vi "main.vi"() -> ()   [LabVIEW 2013]
uses:
  <vilib>/Utility/error.llb/DialogType.ctl
panel:
  out "con status":bool
  in  "Autoscale":bool=TRUE
  in  "P max":dbl=300.0 min=2.0 max=500.0 step=0.1
  in  "P min":dbl=4.0 min=-10.0 max=350.0 step=0.1
  in  "ВКЛ/ВЫКЛ 4":bool=TRUE
  in  "ВКЛ/ВЫКЛ 3":bool=TRUE
  in  "ВКЛ/ВЫКЛ 2":bool
  in  "ВКЛ/ВЫКЛ 1":bool=TRUE
  out "B2":string
  out "B1":string
  out "A2":string
  out "A1":string
  in  "remote port":u16=4001
  in  "address":string="192.168.127.253"
  in  "xScale +":bool
  in  "xScale -":bool
  in  "Добавить время":dbl(ring)=300.0 items=["1 мин."=60.0, "5 мин."=300.0, "20 мин."=1200.0]
  out "мин.":string="1"
  out "часы":string="0"
  out "Graphs hP":dynamicdata(graph) caption="Высокий вакуум, мБар"
  out "сек.":string="0"
  out "Сутки":string
  out "Graphs lP":dynamicdata(graph) caption="Низкий вакуум, мБар"
  in  "stop":bool
  # "Интервал просмотра"
  # ":"
types:
  T1 = typedef "DialogType.ctl" = u16
  T2 = typedef "LVDateTimeRec.ctl" = cluster{"fractional second":dbl, "second":i32, "minute":i32, "hour":i32, "day of month":i32, "month":i32, "year":i32, "day of week":i32, "day of year":i32, "DST":i32}
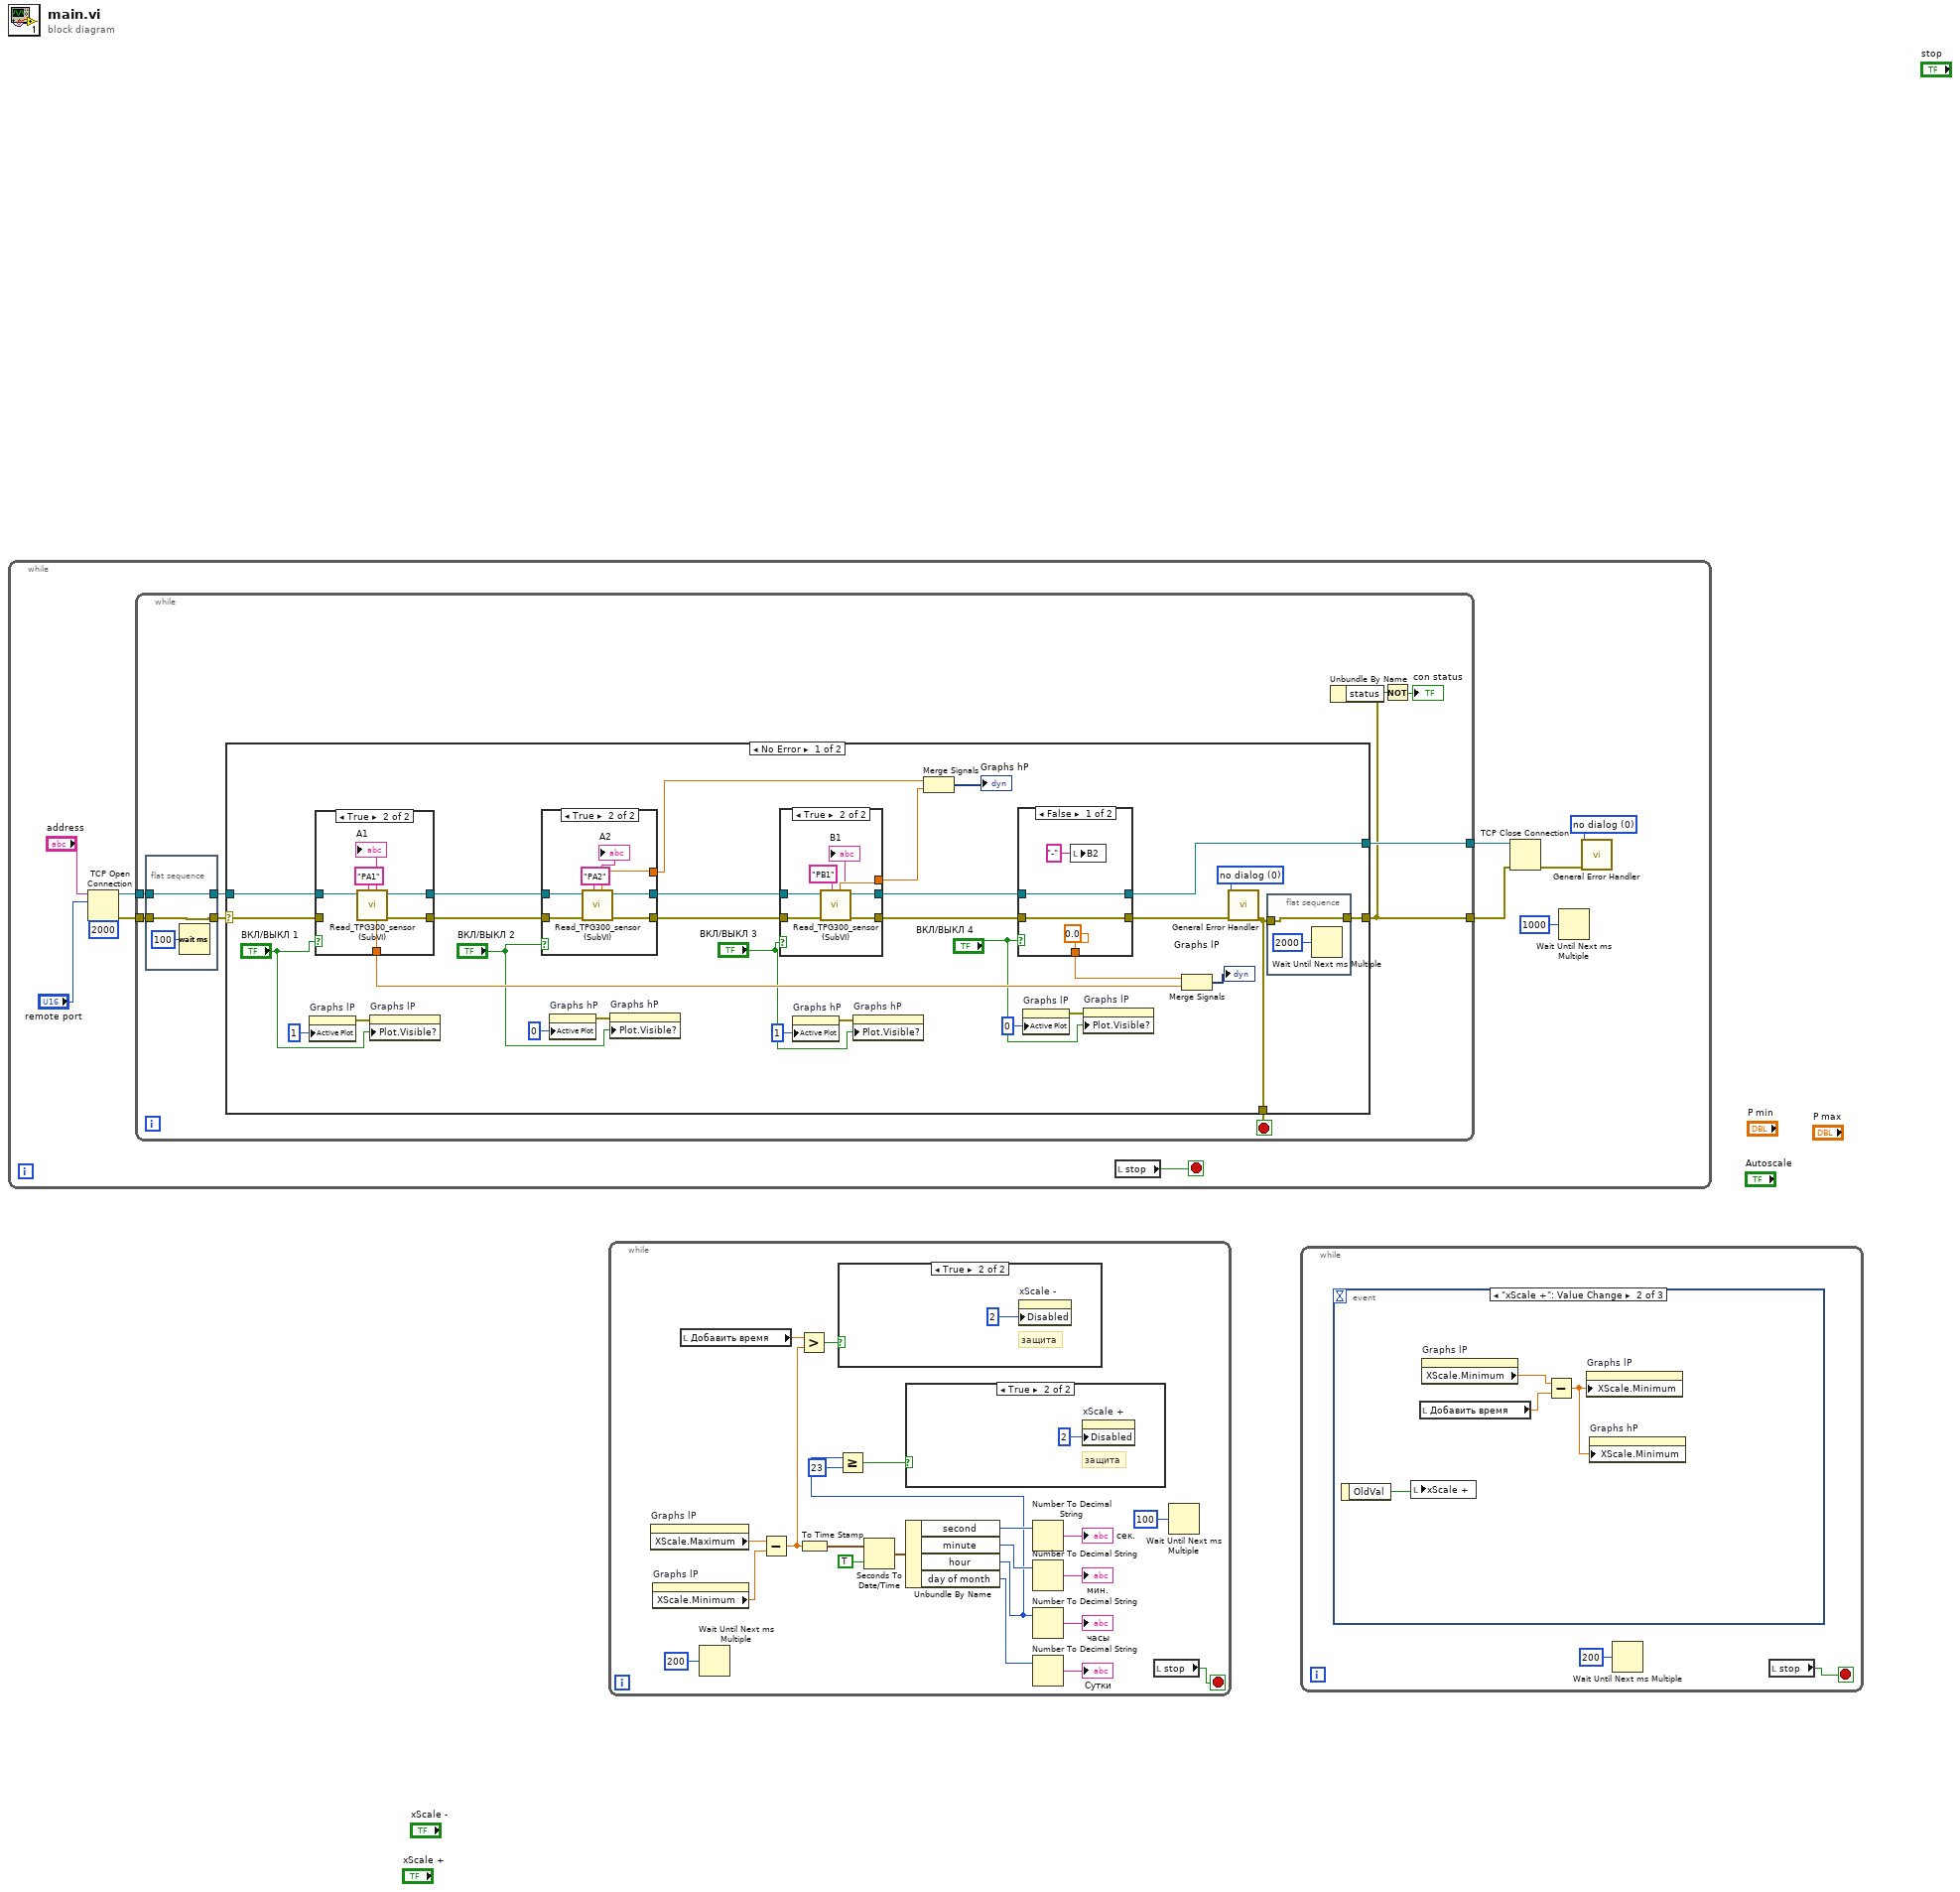
[diagram p0: block diagram]
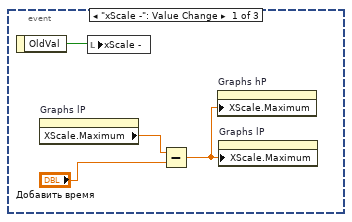
[diagram p2: hidden frame]
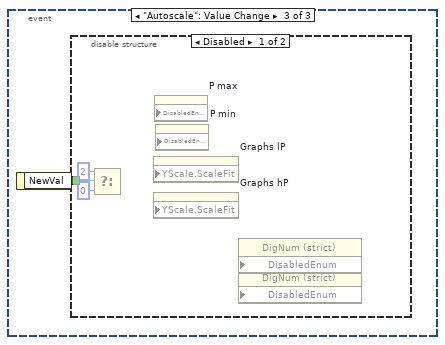
[diagram p3: hidden frame]
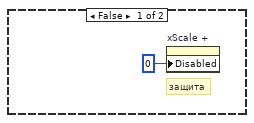
[diagram p5: hidden frame]
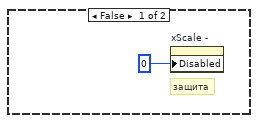
[diagram p6: hidden frame]
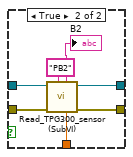
[diagram p7: hidden frame]
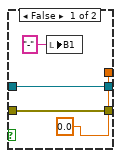
[diagram p8: hidden frame]
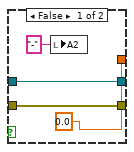
[diagram p9: hidden frame]
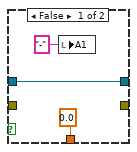
[diagram p10: hidden frame]
diagram:
  n1 = while {
    stop <- w11 stop-if-true
    w5 = T1 0 items=["no dialog", "OK message", "continue or stop message", "OK message + warnings", "continue/stop + warnings"] ("type of dialog (OK msg:1)")
    n2 = TCP Open Connection(address="address", remote port or service name="remote port", timeout ms (60000)=2000) -> (connection ID=w9:refnum<k5>, error out=w8:errorcluster)  [unwired: 1 in, 1 out]
    n3 = while {
      tunnel: w9 -> [w18]
      tunnel: w8 -> [w15]
      tunnel: [w19] -> w6
      tunnel: [w14] -> w3
      stop <- w20 stop-if-true
      n4 = flat-sequence {
        tunnel: w18 -> [w23]
        tunnel: [w23] -> w17
        tunnel: [w22] -> w16
        tunnel: w15 -> [w22]
        frame #0 {
          n5 = Wait (ms)(milliseconds to wait=u32 100) -> ()  [unwired: 1 out]
        }
      }
      n6 = case shown="No Error" w16 {
        selector: w16 -> [w54 w99]
        tunnel: w17 -> [w53 w100]
        tunnel: [w29 w99] -> w20
        tunnel: [w43 w100] -> w19
        tunnel: [w28 w99] -> w14
        frame No Error {
          w44 = T1 0 items=["no dialog", "OK message", "continue or stop message", "OK message + warnings", "continue/stop + warnings"] ("type of dialog (OK msg:1)")
          n7 = property on="Graphs lP" class="WFChart (strict)"("Active Plot"=u32 1) -> (error out=w40:errorcluster)  [unwired: 2 in, 1 out]
          n8 = case shown="True" "ВКЛ/ВЫКЛ 1" {
            tunnel: w54 -> [_ _]
            tunnel: w53 -> [w92 w98]
            tunnel: [_ w96] -> w52
            tunnel: [w92 w95] -> w51
            tunnel: [0.0 ("out number") w94] -> w50
            frame False {
              n9 = local write "A1"("-" ("A1")) -> ()
            }
            frame True {
              n10 = call "Read_TPG300_sensor (SubVI).vi"("Sensor CMD"="PA1" ("data in"), "TCP Network Connection in"=w98) -> ("error out"=w96:errorcluster, "connection ID out"=w95:refnum<k5>, "out number"=w94:dbl, "data out"=→"A1":string)  [unwired: 6 in]
            }
          }
          n11 = property on="Graphs lP" class="WFChart (strict)"(error in=w40, "Plot.Visible?"="ВКЛ/ВЫКЛ 1") -> ()  [unwired: 1 in, 2 out]
          n12 = case shown="True" "ВКЛ/ВЫКЛ 2" {
            tunnel: w52 -> [w81 w89]
            tunnel: w51 -> [w82 w88]
            tunnel: [w82 w87] -> w48
            tunnel: [w81 w86] -> w49
            tunnel: [0.0 ("out number") w84] -> w26
            frame False {
              n13 = local write "A2"("-" ("A2")) -> ()
            }
            frame True {
              n14 = call "Read_TPG300_sensor (SubVI).vi"("Sensor CMD"="PA2" ("data in"), "error in (no error)"=w89, "TCP Network Connection in"=w88) -> ("error out"=w86:errorcluster, "connection ID out"=w87:refnum<k5>, "out number"=w84:dbl, "data out"=→"A2":string)  [unwired: 5 in]
            }
          }
          n15 = property on="Graphs hP" class="WFChart (strict)"("Active Plot"=u32 0) -> (error out=w38:errorcluster)  [unwired: 2 in, 1 out]
          n16 = property on="Graphs hP" class="WFChart (strict)"(error in=w38, "Plot.Visible?"="ВКЛ/ВЫКЛ 2") -> ()  [unwired: 1 in, 2 out]
          n17 = case shown="True" "ВКЛ/ВЫКЛ 3" {
            tunnel: w49 -> [w70 w77]
            tunnel: w48 -> [w71 w76]
            tunnel: [w70 w75] -> w47
            tunnel: [w71 w74] -> w46
            tunnel: [0.0 ("out number") w73] -> w25
            frame False {
              n18 = local write "B1"("-" ("B1")) -> ()
            }
            frame True {
              n19 = call "Read_TPG300_sensor (SubVI).vi"("Sensor CMD"="PB1" ("data in"), "error in (no error)"=w77, "TCP Network Connection in"=w76) -> ("error out"=w75:errorcluster, "connection ID out"=w74:refnum<k5>, "out number"=w73:dbl, "data out"=→"B1":string)  [unwired: 5 in]
            }
          }
          n20 = property on="Graphs hP" class="WFChart (strict)"("Active Plot"=u32 1) -> (error out=w34:errorcluster)  [unwired: 2 in, 1 out]
          n21 = property on="Graphs hP" class="WFChart (strict)"(error in=w34, "Plot.Visible?"="ВКЛ/ВЫКЛ 3") -> ()  [unwired: 1 in, 2 out]
          n22 = Merge Signals(w26, w25) -> (→"Graphs hP":dynamicdata)
          n23 = case shown="False" "ВКЛ/ВЫКЛ 4" {
            tunnel: w47 -> [w60 w66]
            tunnel: w46 -> [w59 w65]
            tunnel: [0.0 ("out number") w64] -> w27
            tunnel: [w60 w63] -> w45
            tunnel: [w59 w62] -> w43
            frame False {
              n24 = local write "B2"("-" ("B2")) -> ()
            }
            frame True {
              n25 = call "Read_TPG300_sensor (SubVI).vi"("Sensor CMD"="PB2" ("data in"), "error in (no error)"=w66, "TCP Network Connection in"=w65) -> ("error out"=w63:errorcluster, "connection ID out"=w62:refnum<k5>, "out number"=w64:dbl, "data out"=→"B2":string)  [unwired: 5 in]
            }
          }
          n26 = property on="Graphs lP" class="WFChart (strict)"("Active Plot"=u32 0) -> (error out=w32:errorcluster)  [unwired: 2 in, 1 out]
          n27 = property on="Graphs lP" class="WFChart (strict)"(error in=w32, "Plot.Visible?"="ВКЛ/ВЫКЛ 4") -> ()  [unwired: 1 in, 2 out]
          n28 = Merge Signals(w27, w50) -> (→"Graphs lP":dynamicdata)
          n29 = call <vilib>:"General Error Handler.vi"("type of dialog (OK msg:1)"=w44, "error in (no error)"=w45) -> ("error out"=w29:errorcluster)  [unwired: 9 in, 4 out]
          n30 = flat-sequence {
            tunnel: w29 -> [w55]
            tunnel: [w55] -> w28
            frame #0 {
              n31 = Wait Until Next ms Multiple(millisecond multiple=u32 2000) -> ()  [unwired: 1 out]
            }
          }
        }
        frame Error {
        }
      }
      n32 = Unbundle By Name(w14) -> ("status"=w13:bool)
      n33 = Not(x=w13) -> (.not. x?=→"con status":bool)
    }
    n34 = local read "stop"() -> (w11:bool)
    n35 = TCP Close Connection(connection ID=w6, error in (no error)=w3) -> (error out=w4:errorcluster)  [unwired: 1 in, 1 out]
    n36 = Wait Until Next ms Multiple(millisecond multiple=u32 1000) -> ()  [unwired: 1 out]
    n37 = call <vilib>:"General Error Handler.vi"("type of dialog (OK msg:1)"=w5, "error in (no error)"=w4) -> ()  [unwired: 9 in, 5 out]
  }
  n38 = while {
    stop <- w102 stop-if-true
    n39 = property on="Graphs lP" class="WFChart (strict)"() -> ("XScale.Maximum"=w121:dbl)  [unwired: 2 in, 2 out]
    n40 = property on="Graphs lP" class="WFChart (strict)"() -> ("XScale.Minimum"=w120:dbl)  [unwired: 2 in, 2 out]
    n41 = local read "Добавить время"() -> (w118:dbl)
    n42 = Wait Until Next ms Multiple(millisecond multiple=u32 200) -> ()  [unwired: 1 out]
    n43 = Subtract(x=w121, y=w120) -> (x-y=w107:dbl)
    n44 = Greater?(x=w118, y=w107) -> (0:w119:bool)
    n45 = To Time Stamp(1:w107) -> (0:w116:timestamp)
    n46 = case shown="True" w119 {
      frame False {
        # "защита"
        n47 = property on="xScale -" class="Bool (strict)"("Disabled"=u8 0) -> ()  [unwired: 2 in, 2 out]
      }
      frame True {
        # "защита"
        n48 = property on="xScale -" class="Bool (strict)"("Disabled"=u8 2) -> ()  [unwired: 2 in, 2 out]
      }
    }
    n49 = Seconds To Date/Time(time stamp (now)=w116, to UTC (F)=TRUE) -> (date time rec=w115:T2)
    n50 = Unbundle By Name(w115) -> ("second"=w114:i32, "minute"=w113:i32, "hour"=w104:i32, "day of month"=w112:i32)
    n51 = Greater Or Equal?(x=w104, y=23) -> (x >= y?=w105:bool)
    n52 = case shown="True" w105 {
      frame False {
        # "защита"
        n53 = property on="xScale +" class="Bool (strict)"("Disabled"=u8 0) -> ()  [unwired: 2 in, 2 out]
      }
      frame True {
        # "защита"
        n54 = property on="xScale +" class="Bool (strict)"("Disabled"=u8 2) -> ()  [unwired: 2 in, 2 out]
      }
    }
    n55 = Number To Decimal String(number=w114) -> (decimal integer string=→"сек.":string)  [unwired: 1 out]
    n56 = Number To Decimal String(number=w113) -> (decimal integer string=→"мин.":string)  [unwired: 1 out]
    n57 = Number To Decimal String(number=w104) -> (decimal integer string=→"часы":string)  [unwired: 1 out]
    n58 = Number To Decimal String(number=w112) -> (decimal integer string=→"Сутки":string)  [unwired: 1 out]
    n59 = local read "stop"() -> (w102:bool)
    n60 = Wait Until Next ms Multiple(millisecond multiple=u32 100) -> ()  [unwired: 1 out]
  }
  n61 = while {
    stop <- w127 stop-if-true
    n62 = event shown="[1] \"xScale +\": Value Change" {
      selector: _ -> [_ _ _]
      dyn-events: _ -> [_ _ _]
      timeout: _ -> [_ _ _]
      event "xScale -": Value Change {
        n63 = event-data() -> ("OldVal"=w131:bool)  [unwired: 1 in]
        n64 = property on="Graphs lP" class="WFChart (strict)"() -> ("XScale.Maximum"=w130:dbl)  [unwired: 2 in, 2 out]
        n65 = local write "xScale -"(w131) -> ()
        n66 = Subtract(x=w130, y="Добавить время") -> (x-y=w128:dbl)
        n67 = property on="Graphs hP" class="WFChart (strict)"("XScale.Maximum"=w128) -> ()  [unwired: 2 in, 2 out]
        n68 = property on="Graphs lP" class="WFChart (strict)"("XScale.Maximum"=w128) -> ()  [unwired: 2 in, 2 out]
      }
      event "xScale +": Value Change {
        n69 = event-data() -> ("OldVal"=w135:bool)  [unwired: 1 in]
        n70 = local write "xScale +"(w135) -> ()
        n71 = local read "Добавить время"() -> (w134:dbl)
        n72 = property on="Graphs lP" class="WFChart (strict)"() -> ("XScale.Minimum"=w133:dbl)  [unwired: 2 in, 2 out]
        n73 = Subtract(x=w133, y=w134) -> (x-y=w132:dbl)
        n74 = property on="Graphs lP" class="WFChart (strict)"("XScale.Minimum"=w132) -> ()  [unwired: 2 in, 2 out]
        n75 = property on="Graphs hP" class="WFChart (strict)"("XScale.Minimum"=w132) -> ()  [unwired: 2 in, 2 out]
      }
      event "Autoscale": Value Change {
        n76 = event-data() -> ("NewVal"=w136:bool)  [unwired: 1 in]
        n77 = disable-structure shown="Disabled" {
          disable-tunnel: w136 -> [w137 _]
          frame Disabled {
            n78 = Select(t=u8 2 ("Y Scale.Scale Fit"), s=w137, f=u8 0 ("Y Scale.Scale Fit")) -> ()  [unwired: 1 out]
            n79 = property on="Graphs lP" class="WFChart (strict)" props=["YScale", "ScaleFit"]() -> ()  [unwired: 3 in, 2 out]
            n80 = property on="Graphs hP" class="WFChart (strict)" props=["YScale", "ScaleFit"]() -> ()  [unwired: 3 in, 2 out]
            n81 = property on="P max" class="DigNum (strict)" props=["DisabledEnum"]() -> ()  [unwired: 3 in, 2 out]
            n82 = property on="P min" class="DigNum (strict)" props=["DisabledEnum"]() -> ()  [unwired: 3 in, 2 out]
            n83 = property on="Property Node" class="DigNum (strict)" props=["DisabledEnum"]() -> ()  [unwired: 3 in, 2 out]
            n84 = property on="Property Node" class="DigNum (strict)" props=["DisabledEnum"]() -> ()  [unwired: 3 in, 2 out]
          }
          frame Enabled {
          }
        }
      }
    }
    n85 = Wait Until Next ms Multiple(millisecond multiple=u32 200) -> ()  [unwired: 1 out]
    n86 = local read "stop"() -> (w127:bool)
  }
